vi "ADI_IMU_ADIS16448_OffsetComp.vi"(6 "error in":errorcluster, 8 "Bytes per Sample":u32, 9 "n Samples":u32=1000) -> (0 "error out":errorcluster, 1 "Sensor Ready?":bool, 2 "Offsets":dbl[](array[numeric]), 3 "Timestamp":u32)   [LabVIEW 2019, in "ADIS16448_IMU.lvlib"]
uses:
  ADIS16448_IMU.lvlib
  <vilib>/Rock Robotics/SystemInterfaces/DIO/FPGA_DIOChannel.ctl
  <vilib>/Analysis/baseanly.llb/Mean (DBL).vi
  <vilib>/Analysis/NI_AALBase.lvlib
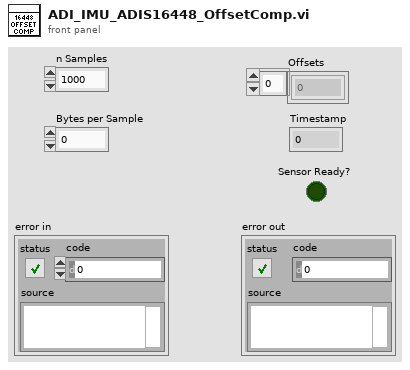
[diagram p1: front panel]
types:
  T1 = typedef "FPGA_DIOChannel.ctl" = enum8{"DIO 0", "DIO 1", "DIO 2", "DIO 3", "DIO 4", "DIO 5", "DIO 6", "DIO 7", "DIO 8", "DIO 9", "DIO MXP 0", "DIO MXP 1", "DIO MXP 2", "DIO MXP 3", "DIO MXP 4", "DIO MXP 5", "DIO MXP 6", "DIO MXP 7", "DIO MXP 8", "DIO MXP 9", "DIO MXP 10", "DIO MXP 11", "DIO MXP 12", "DIO MXP 13", "DIO MXP 14", "DIO MXP 15", "SPI Port CS1", "SPI Port CS2", "SPI Port CS3", "SPI Port MISO", "SPI Port MOSI", "Invalid"}
  T2 = typedef "WPI_DigitalOutputDevRef.ctl" = cluster{"DIO Channel":T1, "DevStatus":errorcluster}
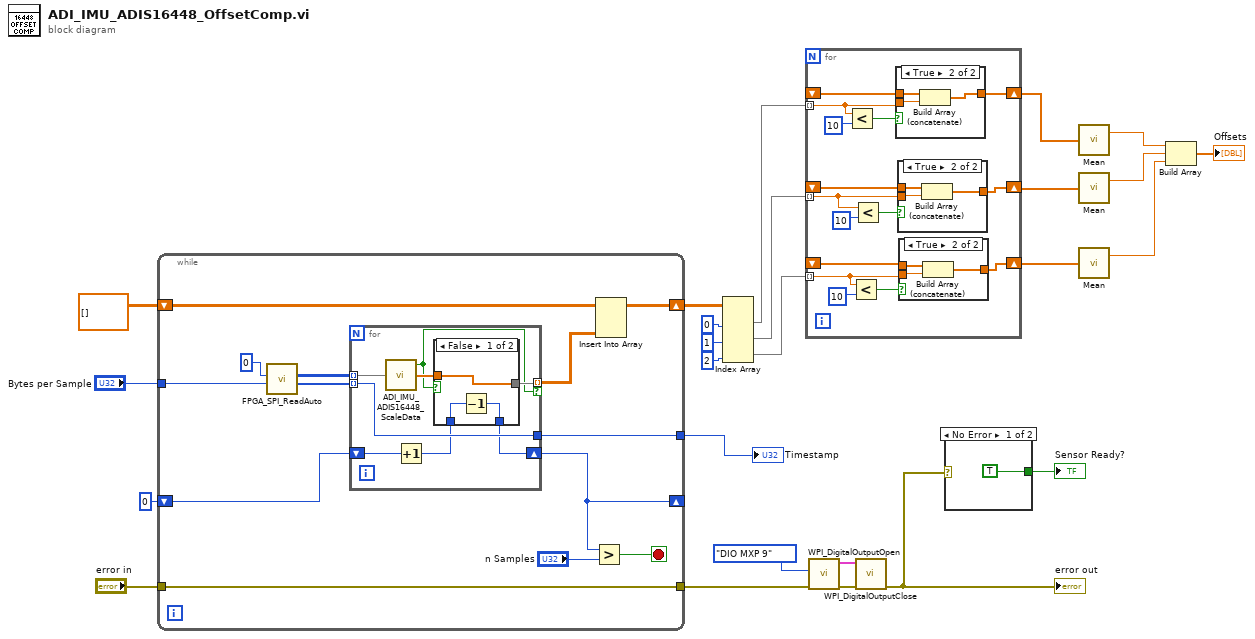
[diagram p0: block diagram]
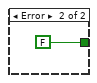
[diagram p5: hidden frame]
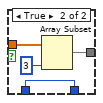
[diagram p6: hidden frame]
diagram:
  n1 = while {
    shift-right: [w34] -> w11
    shift-left: dbl[][] [] -> [w33]
    shift-right: [w28] -> _
    shift-left: u32 0 -> [w29]
    tunnel: "Bytes per Sample" -> [w30]
    tunnel: [w27] -> w19
    tunnel: [w26] -> w15
    tunnel: "error in" -> [w26]
    stop <- w31 stop-if-true
    n2 = call <vilib>:"FPGA_SPI_ReadAuto.vi"("Bytes per Sample"=w30, "Samples to Read"=u32 0) -> ("Timestamps"=w36:u32[], "Data"=w37:u8[][])  [unwired: 7 in, 1 out]
    n3 = for {
      tunnel: w37 -> [w46] mode=indexing
      tunnel: [w44] -> w35 mode=indexing if=w39
      tunnel: w36 -> [w43] mode=indexing
      tunnel: [w43] -> w27
      shift-right: [w40] -> w28
      shift-left: w29 -> [w42]
      n4 = call "ADI_IMU_ADIS16448_ScaleData.vi"("Received Data"=w46) -> ("Data Array"=w45:dbl[], "Data Good?"=w39:bool)  [unwired: 3 in]
      n5 = Increment(x=w42) -> (x+1=w41:u32)
      n6 = case shown="False" w39 {
        tunnel: w45 -> [w49 w53]
        tunnel: [w49 w51] -> w44
        tunnel: w41 -> [w48 w50]
        tunnel: [w47 w50] -> w40
        frame False {
          n7 = Decrement(x=w48) -> (x-1=w47:u32)
        }
        frame True {
          n8 = Array Subset(array=w53, length=3) -> (w51:dbl[])  [unwired: 1 in]
        }
      }
    }
    n9 = Greater?(x=w28, y="n Samples") -> (0:w31:bool)
    n10 = Insert Into Array(array=w33, new element=w35) -> (w34:dbl[][])  [unwired: 2 in]
  }
  "Timestamp" <- w19
  n11 = Index Array(array=w11, index (col) #1=0 ("disabled index (col)"), index (col) #2=1 ("index (col)"), index (col) #3=2 ("index (col)")) -> (element #1=w3:dbl[], element #2=w1:dbl[], element #3=w2:dbl[])  [unwired: 3 in]
  n12 = for {
    tunnel: w2 -> [w54] mode=indexing
    tunnel: w1 -> [w58] mode=indexing
    tunnel: w3 -> [w64] mode=indexing
    shift-right: [w62] -> w4
    shift-left: _ -> [w63]
    shift-right: [w59] -> w6
    shift-left: _ -> [w60]
    shift-right: [w55] -> w5
    shift-left: _ -> [w56]
    n13 = Less?(x=w64, y=10) -> (x < y?=w65:bool)
    n14 = Less?(x=w54, y=10) -> (x < y?=w57:bool)
    n15 = Less?(x=w58, y=10) -> (x < y?=w61:bool)
    n16 = case shown="True" w65 {
      tunnel: w64 -> [_ w78]
      tunnel: w63 -> [w77 w79]
      tunnel: [w77 w80] -> w62
      frame False {
      }
      frame True {
        n17 = Build Array (concatenate)(w79, w78) -> (w80:dbl[])
      }
    }
    n18 = case shown="True" w61 {
      tunnel: w58 -> [_ w74]
      tunnel: w60 -> [w73 w75]
      tunnel: [w73 w76] -> w59
      frame False {
      }
      frame True {
        n19 = Build Array (concatenate)(w75, w74) -> (w76:dbl[])
      }
    }
    n20 = case shown="True" w57 {
      tunnel: w54 -> [_ w70]
      tunnel: w56 -> [w69 w71]
      tunnel: [w69 w72] -> w55
      frame False {
      }
      frame True {
        n21 = Build Array (concatenate)(w71, w70) -> (w72:dbl[])
      }
    }
  }
  n22 = call <vilib>:"WPI_DigitalOutputOpen.vi"("error in (no error)"=w15, "DIO Channel"=FPGA_DIOChannel."DIO MXP 9") -> ("error out"=w17:errorcluster, "DigitalOutputDevRef"=w18:T2)  [unwired: 8 in]
  n23 = call <vilib>:"WPI_DigitalOutputClose.vi"("error in (no error)"=w17, "DigitalOutputDevRef"=w18) -> ("error out"=w13:errorcluster)  [unwired: 9 in]
  "error out" <- w13
  n24 = case shown="No Error" w13 {
    tunnel: [TRUE FALSE] -> w12
    frame No Error {
    }
    frame Error {
    }
  }
  "Sensor Ready?" <- w12
  n25 = call-poly <vilib>:"Mean.vi"("X"=w4) -> ("mean"=w8:dbl)  [unwired: 1 out]
  n26 = call-poly <vilib>:"Mean.vi"("X"=w6) -> ("mean"=w9:dbl)  [unwired: 1 out]
  n27 = call-poly <vilib>:"Mean.vi"("X"=w5) -> ("mean"=w10:dbl)  [unwired: 1 out]
  n28 = Build Array(w8, w9, w10) -> (→"Offsets":dbl[])
